vi "WebPage-Custom-Device.Async.vi"(10 "Parameters":variant, 11 "Process":refnum<class "Process.lvclass">) -> ()   [LabVIEW 2026, in "WebPage Addon Engine.lvlib"]
uses:
  WebPage Addon Engine.lvlib
  <vilib>/NI/NIVS Inline Async API/_VS Inline Async API/Process/Process.lvclass
  Shared/Compiled.Settings.ctl
  <vilib>/NI/NIVS Inline Async API/_VS Inline Async API/Process/Process.lvclass/Process.ctl
  <vilib>/NI/NIVS Inline Async API/_Data Access Engine/Access Type Classes/Read/Read.lvclass/Read.ctl
  <vilib>/NI/NIVS Inline Async API/_Data Access Engine/Data Access Engine/Methods/Read.Data.vi
  <vilib>/NI/NIVS Inline Async API/_VS Inline Async API/Process/Data Member Access/Read Data Access.vi
  <vilib>/NI/NIVS Inline Async API/_VS Inline Async API/Error Handling Process/SubVIs/Error.ConvertArray.vi
  <vilib>/NI/NIVS Inline Async API/_Data Access Engine/Access Type Classes/Read/Read.ProcessData.vi
  <vilib>/NI/NIVS Inline Async API/_Data Access Engine/Data Access Engine/Methods/Read.Lookup.vi
  <vilib>/NI/NIVS Inline Async API/_Data Access Engine/Data Access Engine/Data Access Engine.lvclass
  Shared/WebPage Addon Shared.lvlib
  <vilib>/Utility/SystemLogging/NI_SystemLogging.lvlib
panel:
  out "Values":dbl[](array[numeric])
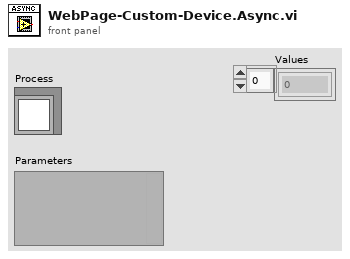
[diagram p1: front panel]
types:
  T1 = typedef "WebPage Addon Shared.lvlib/Compiled.Settings.ctl" = cluster{"Name":string, "Decimation":u32, "Channel Names":string[], "Hosted IP Address":string, "Hosted Port":u32, "gRPC Port":u32}
  T2 = typedef "Data Access Engine.lvlib/Data Access Engine.lvclass/Read.DVR.ctl" = refnum<data-value>
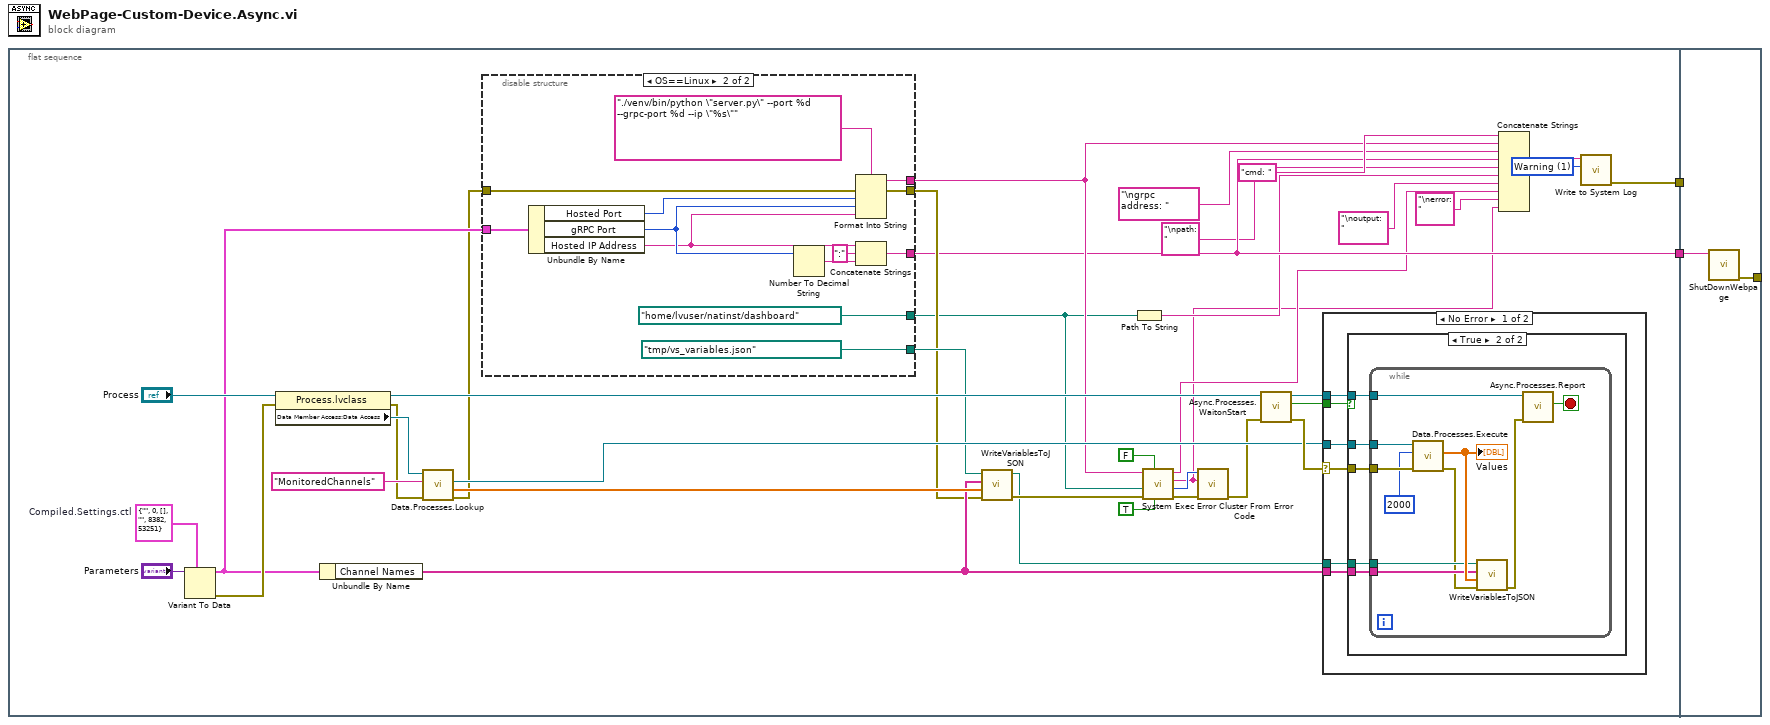
[diagram p0: block diagram]
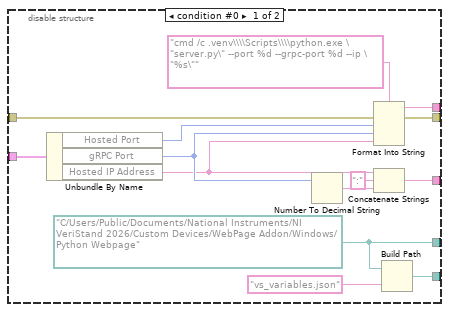
[diagram p2: hidden frame]
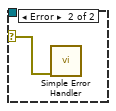
[diagram p4: hidden frame]
diagram:
  n1 = flat-sequence {
    tunnel: [w13] -> w2
    tunnel: [w3] -> w1
    tunnel: [w92] -> _
    tunnel: w2 -> [w91]
    tunnel: w1 -> [_]
    frame #0 {
      w4 = 1 items=["Error", "Warning", "Informational"] ("severity")
      w33 = T1 {"Name"="", "Decimation"=0, "Channel Names"=[], "Hosted IP Address"="", "Hosted Port"=8382, "gRPC Port"=53251}  # Compiled.Settings.ctl
      n2 = Variant To Data(type=w33, Variant="Parameters") -> (data=w19:T1, error out=w32:errorcluster)  [unwired: 1 in]
      n3 = property class="Process.lvclass"(reference="Process", error in=w32) -> (reference out=w36:refnum<class "Process.lvclass">, error out=w25:errorcluster, "Data Member Access:Data Access"=w35:refnum<class "Data Access Engine.lvclass">)
      n4 = Unbundle By Name(w19) -> ("Channel Names"=w22:string[])
      n5 = call-poly <vilib>:"Data.Processes.Lookup.vi"("error in (no error)"=w25, "Name"="MonitoredChannels", "Data Access API in"=w35) -> ("error out"=w18:errorcluster, "Initial Values"=w24:dbl[], "Ref"=w38:T2)  [unwired: 5 in, 1 out]
      n6 = disable-structure shown="OS==Linux" {
        disable-tunnel: [w51 w57] -> w15
        disable-tunnel: [w55 path "/home/lvuser/natinst/dashboard" ("working directory")] -> w11
        disable-tunnel: [w54 path "/tmp/vs_variables.json" ("path")] -> w27
        disable-tunnel: w19 -> [w50 w60]
        disable-tunnel: [w44 w56] -> w13
        disable-tunnel: w18 -> [w43 w61]
        disable-tunnel: [w42 w59] -> w17
        frame condition #0 {
          w55 = path "C:/Users/Public/Documents/National Instruments/NI VeriStand 2026/Custom Devices/WebPage Addon/Windows/Python Webpage" ("working directory")
          n7 = Unbundle By Name(w50) -> ("Hosted Port"=w49:u32, "gRPC Port"=w48:u32, "Hosted IP Address"=w47:string)
          n8 = Number To Decimal String(number=w48) -> (decimal integer string=w46:string)  [unwired: 1 in]
          n9 = Format Into String(format string="cmd /c .venv\\\\Scripts\\\\python.exe \"server.py\" --port %d --grpc-port %d --ip \"%s\"" ("command line"), error in=w43, w49, w48, w47) -> (resulting string=w51:string, error out=w42:errorcluster)  [unwired: 1 in]
          n10 = Concatenate Strings(w47, ":" ("string"), w46) -> (w44:string)
          n11 = Build Path(base path=w55, name or relative path="vs_variables.json" ("command line")) -> (appended path=w54:path)
        }
        frame condition #1 (active) {
          n12 = Unbundle By Name(w60) -> ("Hosted Port"=w66:u32, "gRPC Port"=w65:u32, "Hosted IP Address"=w64:string)
          n13 = Number To Decimal String(number=w65) -> (decimal integer string=w63:string)  [unwired: 1 in]
          n14 = Format Into String(format string="./venv/bin/python \"server.py\" --port %d --grpc-port %d --ip \"%s\"" ("command line"), error in=w61, w66, w65, w64) -> (resulting string=w57:string, error out=w59:errorcluster)  [unwired: 1 in]
          n15 = Concatenate Strings(w64, ":" ("string"), w63) -> (w56:string)
        }
      }
      n16 = call "WriteVariablesToJSON.vi"("error in"=w17, "Channel Values"=w24, "Channel Names"=w22, "path"=w27) -> ("error out"=w26:errorcluster, "path out"=w21:path)  [unwired: 6 in]
      n17 = Path To String(path=w11) -> (string=w10:string)
      n18 = call <vilib>:"System Exec.vi"("run minimized? (F)"=TRUE, "wait until completion? (T)"=FALSE, "error in (no error)"=w26, "working directory"=w11, "command line"=w15) -> ("error out"=w28:errorcluster, "return code"=w29:i32, "standard error"=w6:string, "standard output"=w8:string)  [unwired: 3 in]
      n19 = call <vilib>:"Error Cluster From Error Code.vi"("error in (no error)"=w28, "error message (\"\")"=w6, "error code (0)"=w29) -> ("error out"=w23:errorcluster)  [unwired: 6 in]
      n20 = call <vilib>:"Async.Processes.WaitonStart.vi"("error in (no error)"=w23, "Process"=w36) -> ("error out"=w39:errorcluster, "Execute"=w41:bool, "Process out"=w40:refnum<class "Process.lvclass">)  [unwired: 7 in]
      n21 = case shown="No Error" w39 {
        selector: w39 -> [w71 w90]
        tunnel: w41 -> [w74 _]
        tunnel: w40 -> [w73 _]
        tunnel: w38 -> [w72 _]
        tunnel: w22 -> [w70 _]
        tunnel: w21 -> [w69 _]
        frame No Error {
          n22 = case shown="True" w74 {
            tunnel: w71 -> [_ w77]
            tunnel: w73 -> [_ w78]
            tunnel: w72 -> [_ w79]
            tunnel: w70 -> [_ w76]
            tunnel: w69 -> [_ w75]
            frame False {
            }
            frame True {
              n23 = while {
                tunnel: w77 -> [w86]
                tunnel: w78 -> [w89]
                tunnel: w79 -> [w87]
                tunnel: w76 -> [w83]
                tunnel: w75 -> [w82]
                stop <- w88 stop-if-true
                n24 = call-poly <vilib>:"Data.Processes.Execute.vi"("error in (no error)"=w86, "timeout ms"=2000, "Ref"=w87) -> ("error out"=w81:errorcluster, "Values"=w84:dbl[])  [unwired: 6 in, 1 out]
                "Values" <- w84
                n25 = call "WriteVariablesToJSON.vi"("error in"=w81, "Channel Values"=w84, "Channel Names"=w83, "path"=w82) -> ("error out"=w80:errorcluster)  [unwired: 6 in, 1 out]
                n26 = call <vilib>:"Async.Processes.Report.vi"("Error"=w80, "Process in"=w89) -> ("Stop"=w88:bool)  [unwired: 8 in, 1 out]
              }
            }
          }
        }
        frame Error {
          n27 = call <vilib>:"Simple Error Handler.vi"("error in (no error)"=w90) -> ()  [unwired: 4 in, 5 out]
        }
      }
      n28 = Concatenate Strings("cmd: " ("string"), w15, "\ngrpc address: " ("string"), w13, "\npath: " ("string"), w10, "\noutput: " ("string"), w8, "\nerror: " ("string"), w6) -> (w5:string)
      n29 = call <vilib>:"Write to System Log.vi"("severity"=w4, "message"=w5) -> ("error out"=w3:errorcluster)  [unwired: 9 in]
    }
    frame #1 {
      n30 = call "ShutDownWebpage.vi"("address"=w91) -> ("error out"=w92:errorcluster)  [unwired: 10 in]
    }
  }
